vi "Rinocloud_explorer_subVI.vi"() -> ()   [LabVIEW 2013]
uses:
  Rinocloud Library.lvlib
  Rinocloud_global_variable.vi
  Rinocloud API endpoint VIs/API_endpoint_subVIs/State_Control.ctl
panel:
  in  "System state":T1={"Active items"={"Active file ID"="", "Active dir ID"="", "Active object ID"="", "Recent ID"="", "Active item:"="<folder> home (id=)", "Source item"="", "Destination item"="", "Source ID"="", "Destination ID"=""}, "Trees"={"Ancestors"=refnum, "Children"=refnum, "Metadata"=refnum}, "New metadata"={"Name"="", "Tags"="", "Notes"="", "Custom metadata"=[]}, "Communication"={"HTTP headers"="", "HTTP body"="", "Project name"="", "User"="", "HTTP ch body"=""}, "Controls"={"Move refnum"=refnum}, "Status messages"={"error "={"status"=FALSE, "code"=0, "source"=""}, "status"=""}, "Update metadata"={"Name"="", "Tags"="", "Notes"=""}, "Pagination"={"total"=0.0, "limit"=0.0, "offset"=0.0, "count"=0.0, " next page refnum"=refnum, "previous page refnum"=refnum, "page indicator"=""}} {"New metadata"."Custom metadata"."Data type" items=["Numeric", "String", "1D array of strings", "1D array of doubles", "Data JSON string", "<null>"]}
  in  "Rino status control":T2={"Navigation controls"={"full path tree"=refnum, "folder content tree"=refnum, "next page"=refnum, "previous page"=refnum, "refresh file list"=refnum, "delete"=refnum, "page indicator string"=refnum}, "New Folder controls"={"next folder"=refnum, "name"="", "tags"="", "notes"="", "metadata array"=[]}, "Upload File controls"={"upoad file"=refnum, "name"="", "tags"="", "notes"="", "metadata array"=[], "Store data locally"=TRUE, "Store metadata locally"=FALSE, "Path Refnum"=refnum}, "Metadata management controls"={"get metadata"=refnum, "update metadata"=refnum, "name"=refnum, "tags"=refnum, "notes"=refnum, "metadata tree"=refnum}, "Status indicators"={"error"=refnum, "active item"=refnum, "last action"=refnum, "http header"=refnum, "http body"=refnum}, "Move file controls"={"source item"=refnum, "destination item"=refnum, "set source"=refnum, "set destination"=refnum, "move"=refnum}} {"Upload File controls"."metadata array"."Data type" items=["Numeric", "String", "1D array of strings", "1D array of doubles", "Data JSON string", "<null>"]; "New Folder controls"."metadata array"."Data type" items=["Numeric", "String", "1D array of strings", "1D array of doubles", "Data JSON string", "<null>"]}
  in  "page indicator":string
  in  "Next page":bool
  in  "Previous page":bool
  out "Last action:":string
  in  "Active item:":string="<folder> home (id=)"
  in  "delete":bool
  in  "refresh list":bool
  in  "Tab Control":T3(tab)=enum."Inspect"
  in  "Cluster 2":T4={"Attribute"="", "Value"="", "Data type"=5} {"Data type" items=["Numeric", "String", "1D array of strings", "1D array of doubles", "Data JSON string", "<null>"]}
  in  "Cluster 1":T4={"Attribute"="", "Value"="", "Data type"=5} {"Data type" items=["Numeric", "String", "1D array of strings", "1D array of doubles", "Data JSON string", "<null>"]}
  in  "name":string
  in  "tags":string
  in  "notes":string
  in  "new folder":bool
  in  "upload file":bool
  in  "Store data locally":bool=TRUE
  in  "Store metadata locally":bool
  in  "Name:":string
  in  "Tags:":string
  in  "Notes:":string
  in  "get metadata":bool
  in  "metadata tree":string(tree) caption="Metadata"
  in  "update metadata":bool
  in  "Move":bool
  in  "Destination:":string
  in  "Source:":string
  in  "set source":bool
  in  "set destination":bool
  out "body":string
  out "headers":string
  in  "error message":string caption="Error:"
  in  "ancestor tree":string(tree)="home" caption="Active path"
  in  "stop":bool
  in  "active child tree":string(tree) caption="File & folder list of the active folder"
  # "Double-click an item to activate"
  # "Custom metadata:"
  # "(tag1,tag2,tag3,...)"
  # "Click the fields to edit"
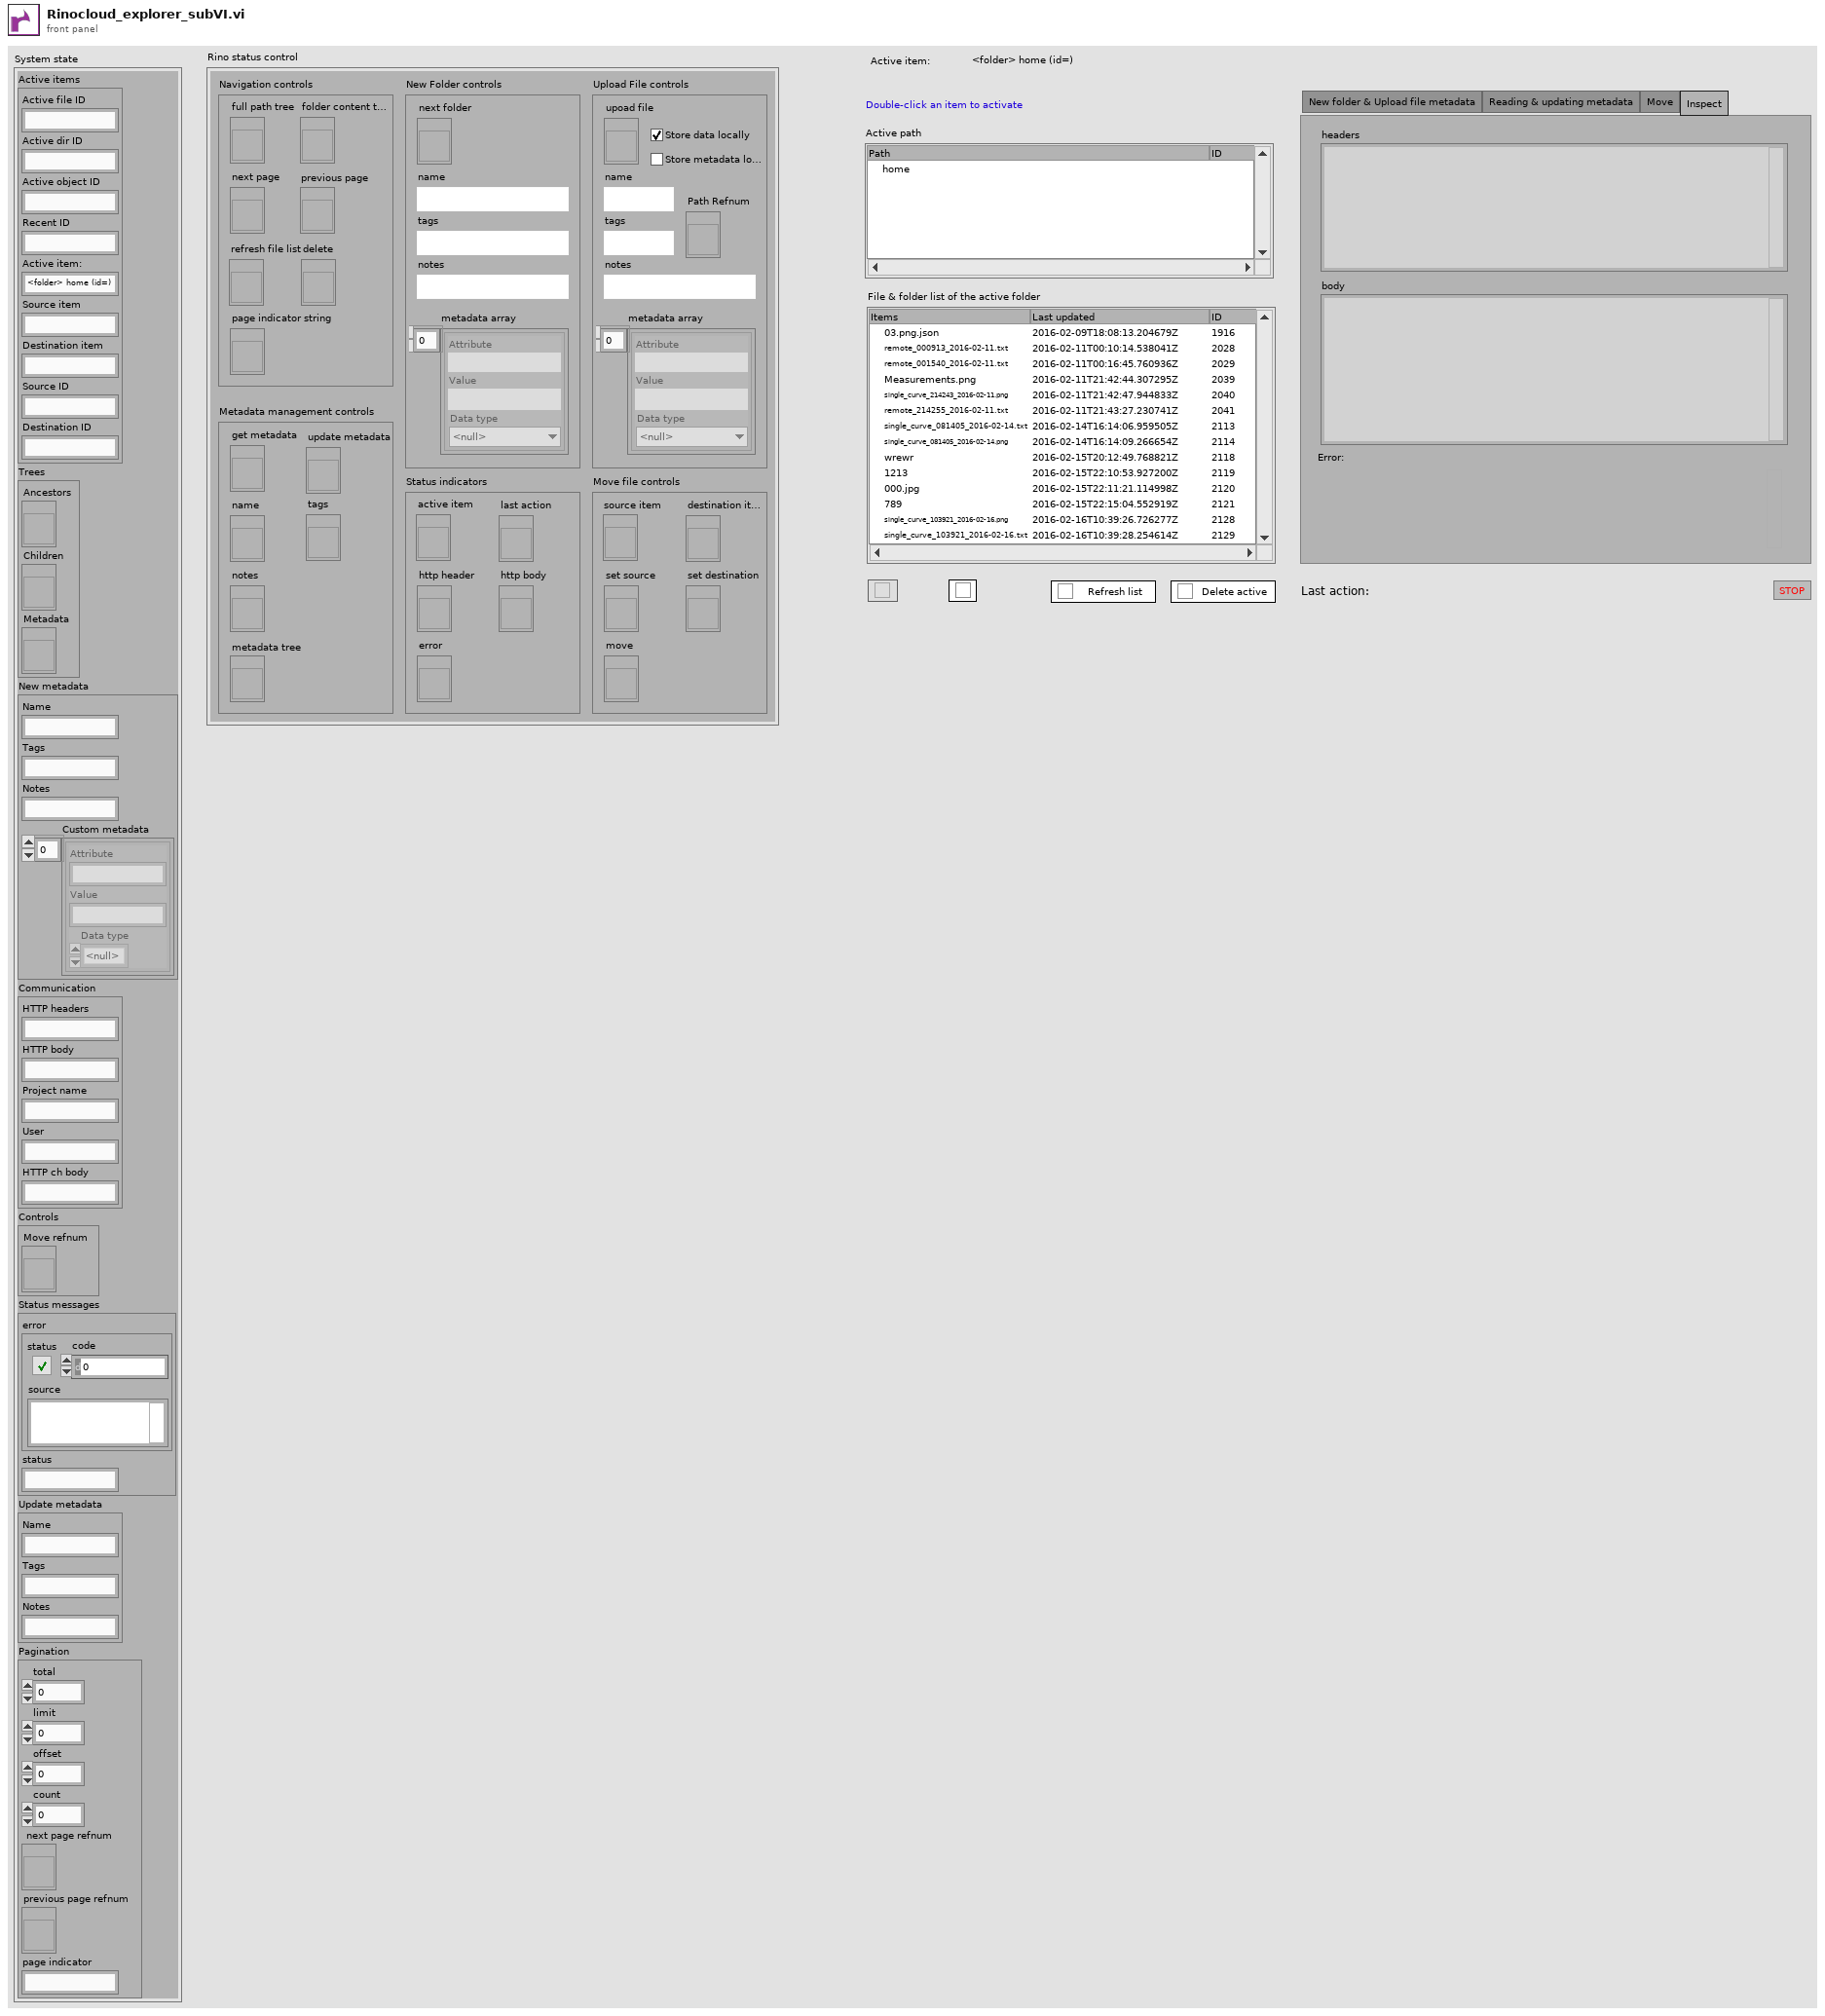
[diagram p1: front panel]
types:
  T1 = cluster{"Active items":cluster{"Active file ID":string, "Active dir ID":string, "Active object ID":string, "Recent ID":string, "Active item:":string, "Source item":string, "Destination item":string, "Source ID":string, "Destination ID":string}, "Trees":cluster{"Ancestors":refnum<vi>, "Children":refnum<vi>, "Metadata":refnum<vi>}, "New metadata":cluster{"Name":string, "Tags":string, "Notes":string, "Custom metadata":cluster{"Attribute":string, "Value":string, "Data type":u16}[]}, "Communication":cluster{"HTTP headers":string, "HTTP body":string, "Project name":string, "User":string, "HTTP ch body":string}, "Controls":cluster{"Move refnum":refnum<vi>}, "Status messages":cluster{"error ":errorcluster, "status":string}, "Update metadata":cluster{"Name":string, "Tags":string, "Notes":string}, "Pagination":cluster{"total":dbl, "limit":dbl, "offset":dbl, "count":dbl, " next page refnum":refnum<vi>, "previous page refnum":refnum<vi>, "page indicator":string}}
  T2 = cluster{"Navigation controls":cluster{"full path tree":refnum<vi>, "folder content tree":refnum<vi>, "next page":refnum<vi>, "previous page":refnum<vi>, "refresh file list":refnum<vi>, "delete":refnum<vi>, "page indicator string":refnum<vi>}, "New Folder controls":cluster{"next folder":refnum<vi>, "name":string, "tags":string, "notes":string, "metadata array":cluster{"Attribute":string, "Value":string, "Data type":u16}[]}, "Upload File controls":cluster{"upoad file":refnum<vi>, "name":string, "tags":string, "notes":string, "metadata array":cluster{"Attribute":string, "Value":string, "Data type":u16}[], "Store data locally":bool, "Store metadata locally":bool, "Path Refnum":refnum<vi>}, "Metadata management controls":cluster{"get metadata":refnum<vi>, "update metadata":refnum<vi>, "name":refnum<vi>, "tags":refnum<vi>, "notes":refnum<vi>, "metadata tree":refnum<vi>}, "Status indicators":cluster{"error":refnum<vi>, "active item":refnum<vi>, "last action":refnum<vi>, "http header":refnum<vi>, "http body":refnum<vi>}, "Move file controls":cluster{"source item":refnum<vi>, "destination item":refnum<vi>, "set source":refnum<vi>, "set destination":refnum<vi>, "move":refnum<vi>}}
  T3 = enum32{"New folder & Upload file metadata", "Reading & updating metadata", "Move", "Inspect"}
  T4 = cluster{"Attribute":string, "Value":string, "Data type":u16}
  T5 = typedef "State_Control.ctl" = enum16{"Boot", "Initialize", "Wait for event", "Refresh", "Pagination", "Metadata to tree", "Stop"}
  T6 = cluster{"HTTP headers":string, "HTTP body":string, "Project name":string, "User":string, "HTTP ch body":string}
  T7 = cluster{"Active file ID":string, "Active dir ID":string, "Active object ID":string, "Recent ID":string, "Active item:":string, "Source item":string, "Destination item":string, "Source ID":string, "Destination ID":string}
  T8 = enum8{"Enabled", "Disabled", "Disabled and Grayed Out"}
  T9 = cluster{"Name":string, "Tags":string, "Notes":string, "Custom metadata":cluster{"Attribute":string, "Value":string, "Data type":u16}[]}
  T10 = enum16{"Boot", "Initialize", "Wait for event", "Refresh", "Pagination", "Metadata to tree", "Stop"}
  T11 = cluster{"Store locally":bool, "ancestor array":cluster{"id":string, "name":string, "created_on":string, "updated_on":string, "tags":string, "notes":string, "record type":string, "metadata (JSON)":string}[], "Store metadata":bool}
  T12 = cluster{"Attribute":string, "Value":string, "Data type":enum16{"Numeric", "String", "1D array of strings", "1D array of doubles", "Data JSON string", "<null>"}}[]
  T13 = cluster{"limit":dbl, "total":dbl, "offset":dbl, "count":dbl}
  T14 = cluster{"headers":string, "body":string, "ID":string, "Saved":bool}
  T15 = cluster{"Attribute":string, "Value":string, "Data type":u16}[]
  T16 = cluster{"id":string, "name":string, "created_on":string, "updated_on":string, "tags":string, "notes":string, "record type":string, "metadata (JSON)":string}[]
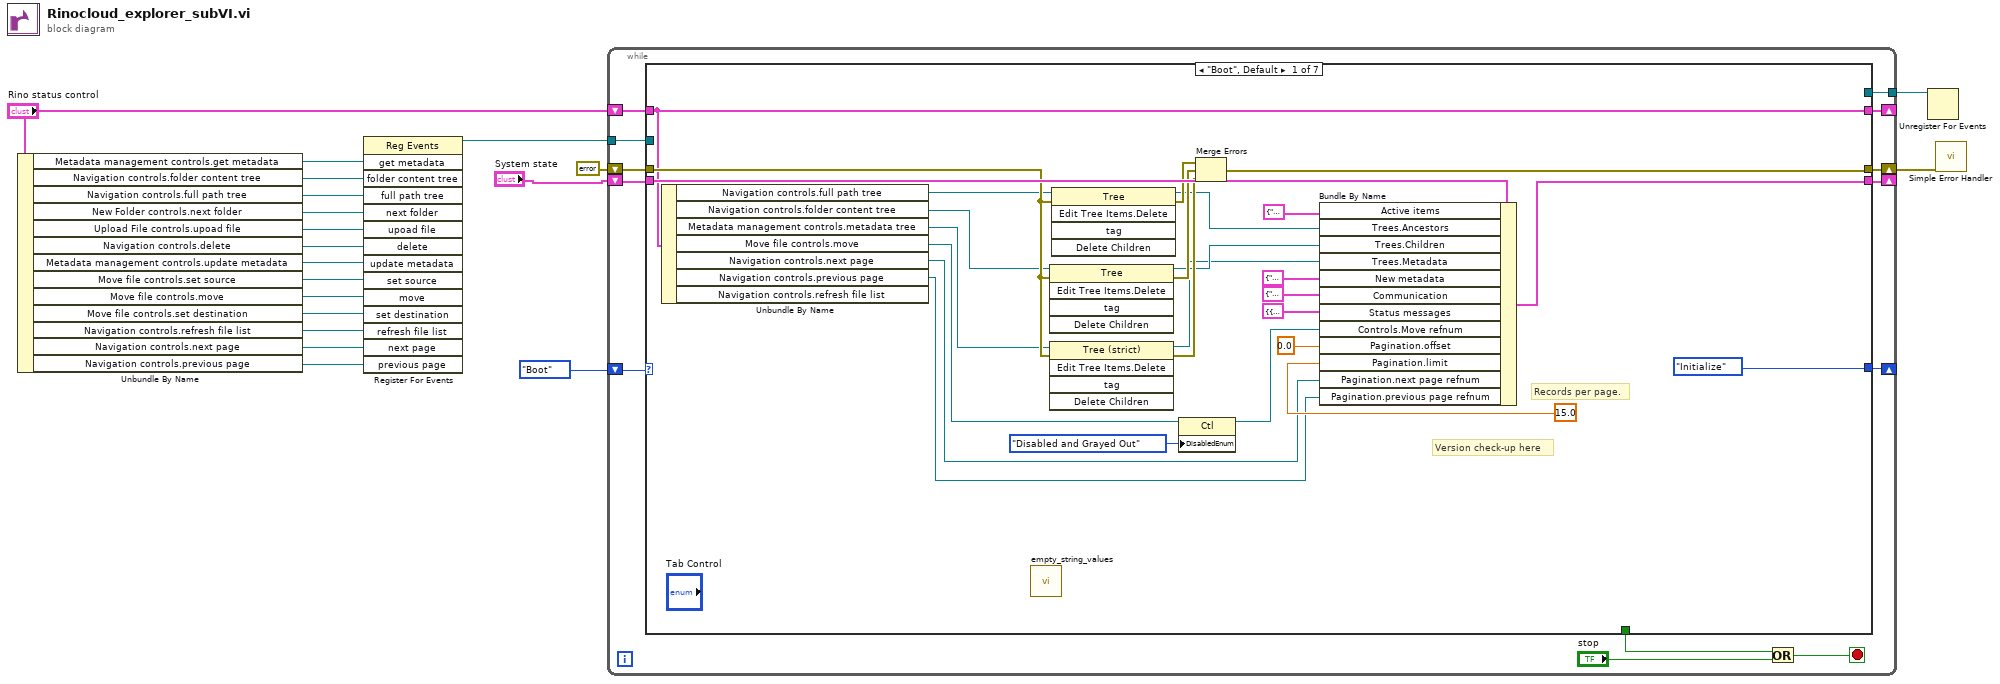
[diagram p0: block diagram]
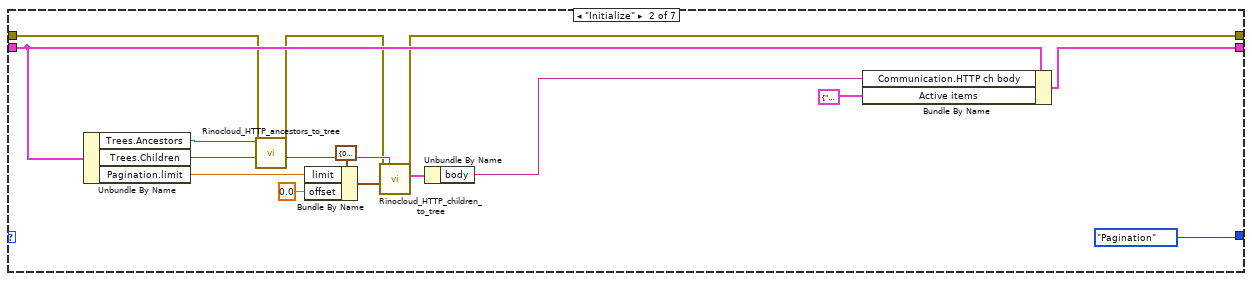
[diagram p2: hidden frame]
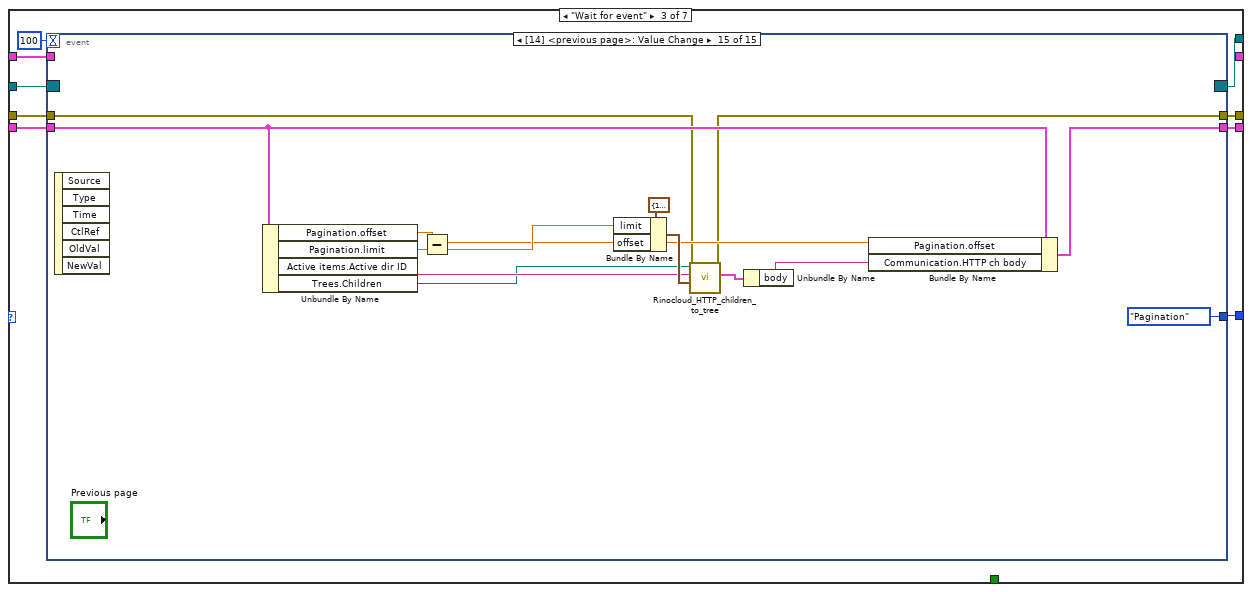
[diagram p3: hidden frame]
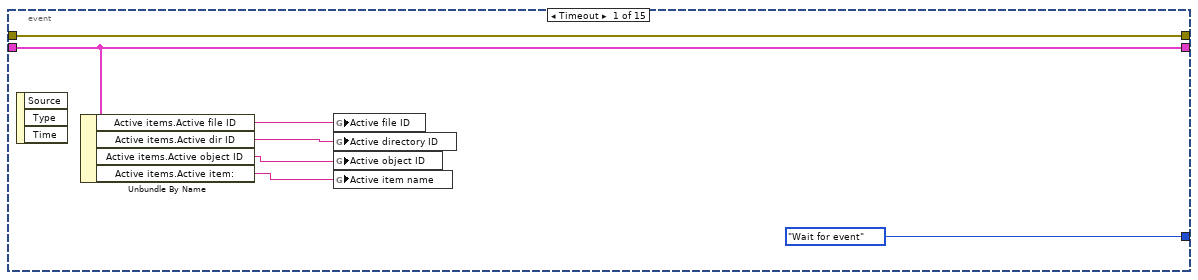
[diagram p4: hidden frame]
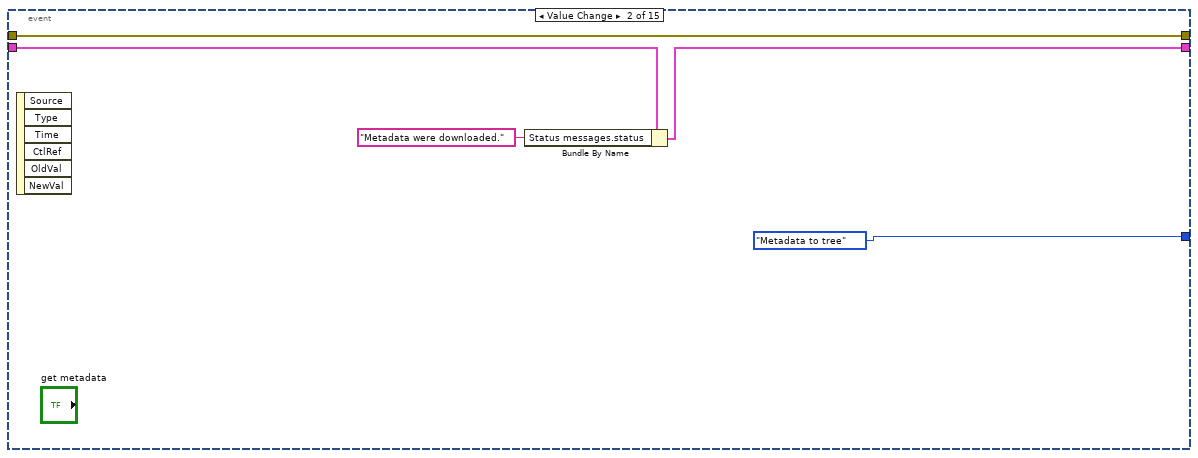
[diagram p5: hidden frame]
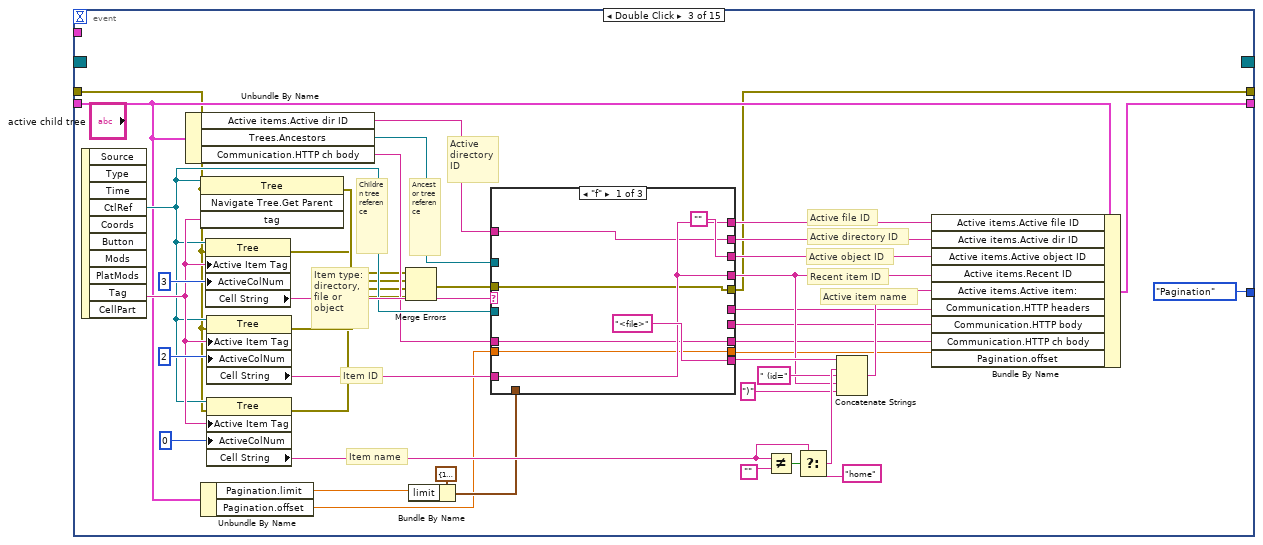
[diagram p6: hidden frame]
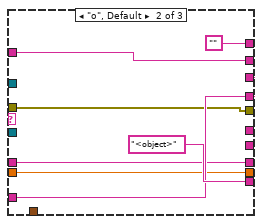
[diagram p7: hidden frame]
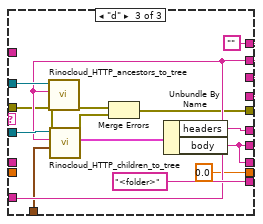
[diagram p8: hidden frame]
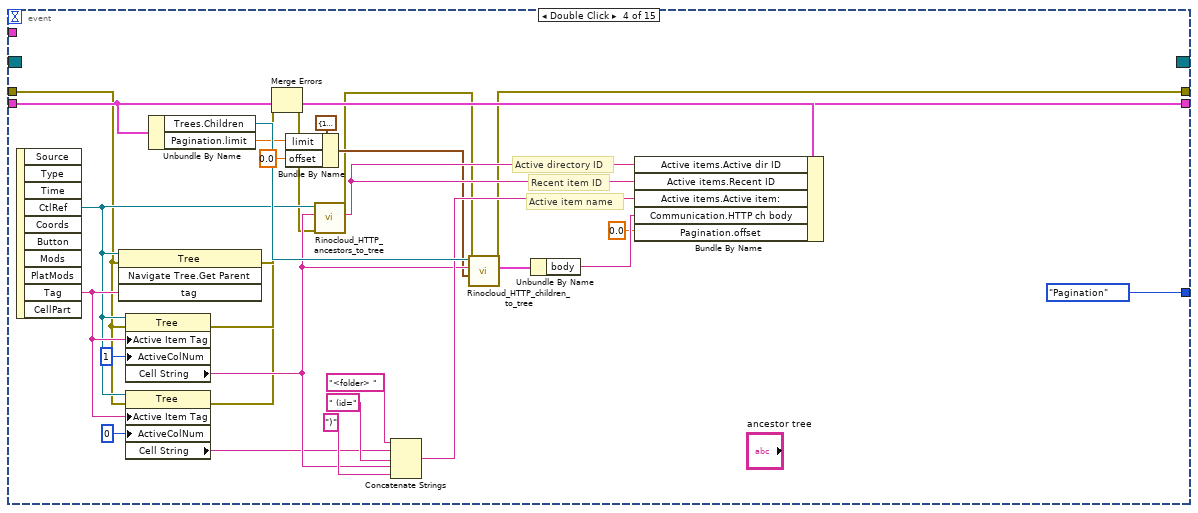
[diagram p9: hidden frame]
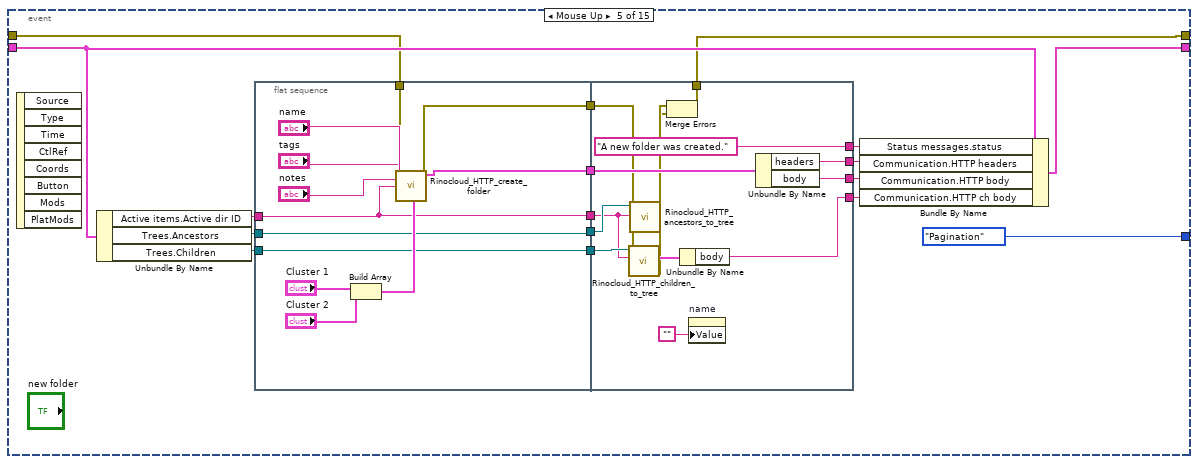
[diagram p10: hidden frame]
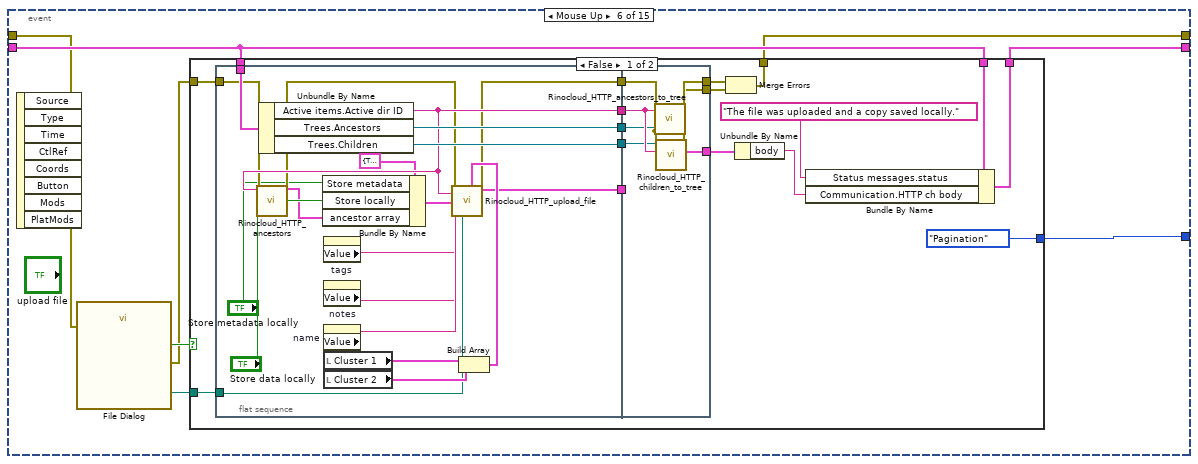
[diagram p11: hidden frame]
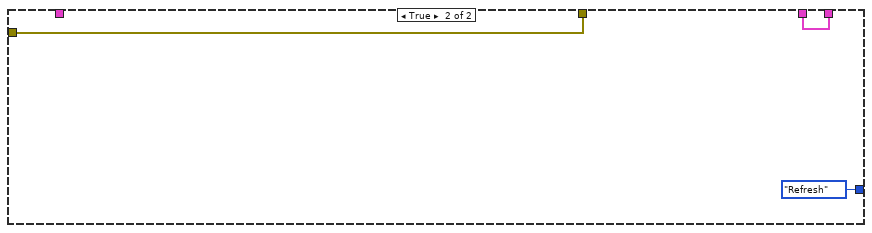
[diagram p12: hidden frame]
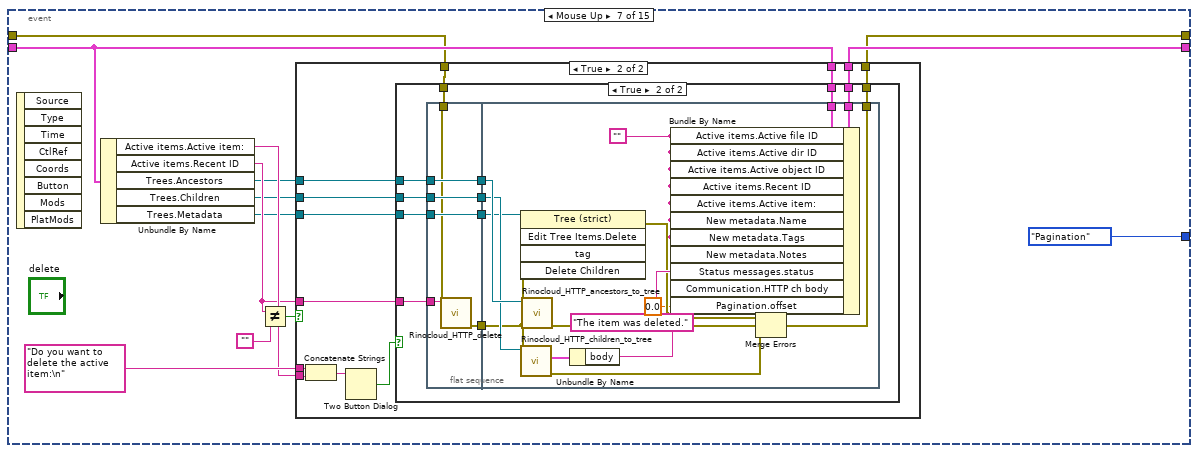
[diagram p13: hidden frame]
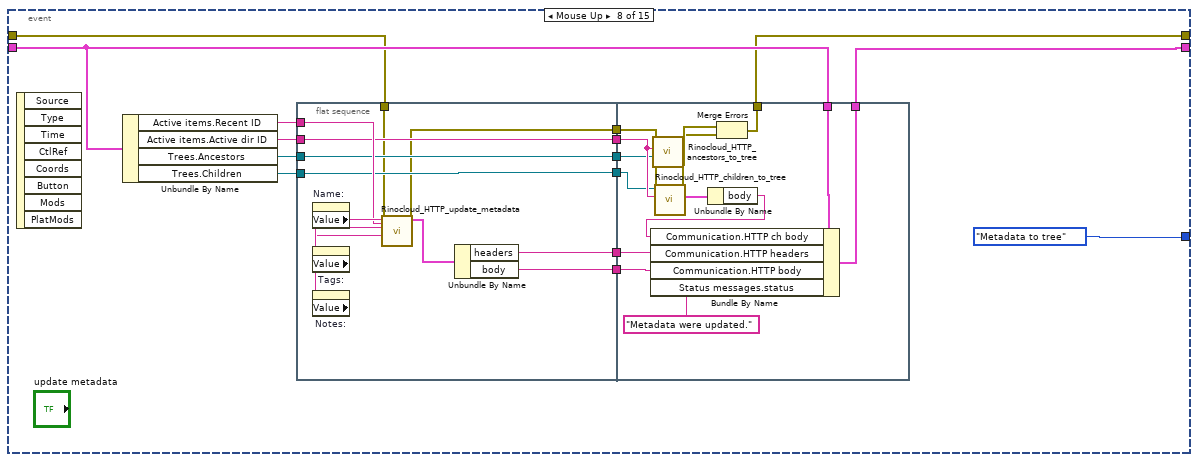
[diagram p16: hidden frame]
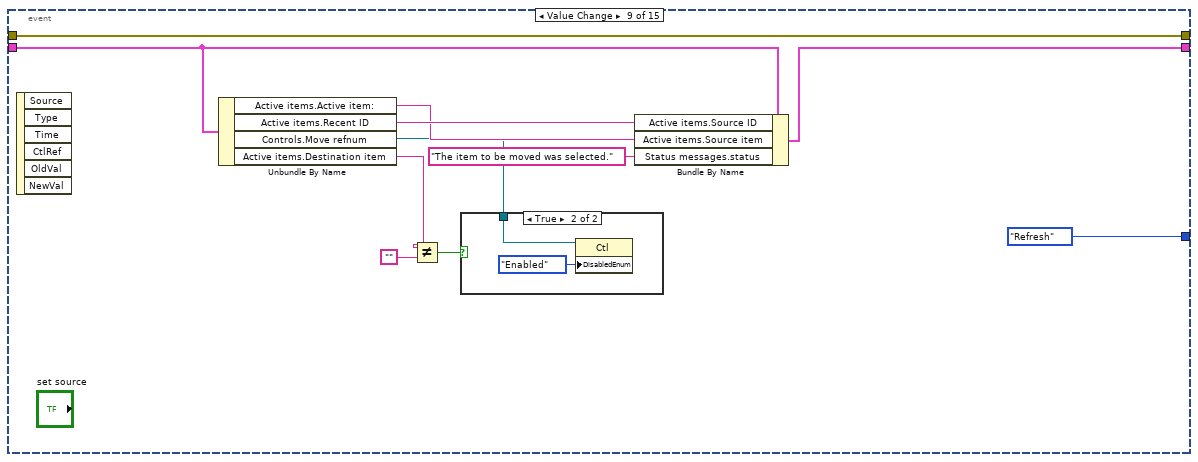
[diagram p17: hidden frame]
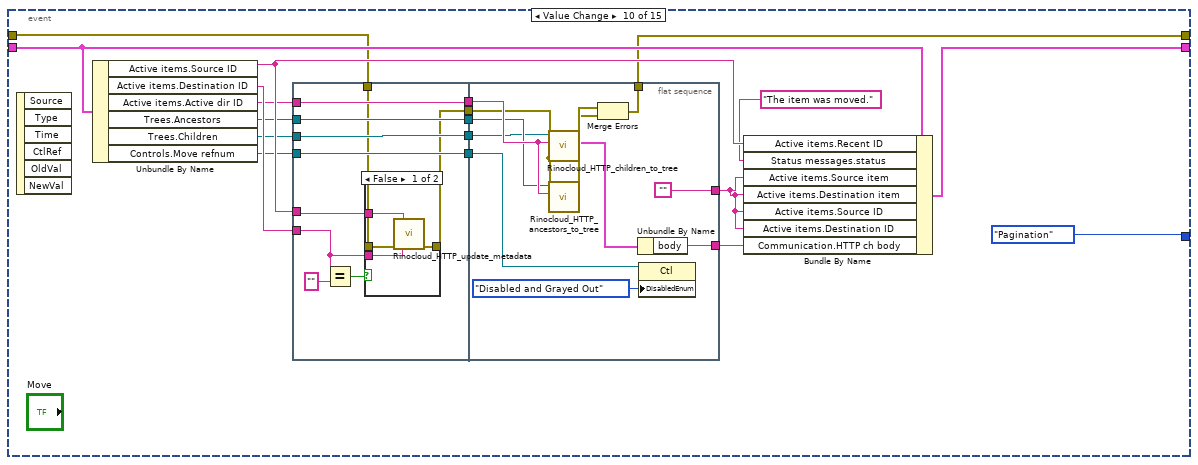
[diagram p19: hidden frame]
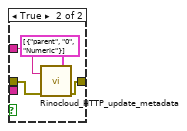
[diagram p20: hidden frame]
diagram:
  n1 = Unbundle By Name("Rino status control") -> ("Metadata management controls.get metadata"=w15:refnum<vi>, "Navigation controls.folder content tree"=w13:refnum<vi>, "Navigation controls.full path tree"=w12:refnum<vi>, "New Folder controls.next folder"=w11:refnum<vi>, "Upload File controls.upoad file"=w10:refnum<vi>, "Navigation controls.delete"=w9:refnum<vi>, "Metadata management controls.update metadata"=w8:refnum<vi>, "Move file controls.set source"=w7:refnum<vi>, "Move file controls.move"=w6:refnum<vi>, "Move file controls.set destination"=w5:refnum<vi>, "Navigation controls.refresh file list"=w4:refnum<vi>, "Navigation controls.next page"=w3:refnum<vi>, "Navigation controls.previous page"=w2:refnum<vi>)
  n2 = register-events(w15, w13, w12, w11, w10, w9, w8, w7, w6, w5, w4, w3, w2) -> (reference out=w17:refnum<event-registration>)  [unwired: 2 in, 1 out]
  n3 = while {
    shift-right: [w27] -> _
    shift-left: State_Control."Boot" -> [w33]
    shift-right: [w28] -> _
    shift-left: "System state" -> [w29]
    shift-right: [w25] -> w18
    shift-left: errorcluster {"status"=FALSE, "code"=0, "source"=""} ("errors") -> [w26]
    tunnel: w17 -> [w24]
    tunnel: [w22] -> w14
    shift-right: [w21] -> _
    shift-left: "Rino status control" -> [w23]
    stop <- w32 stop-if-true
    n4 = case shown="\"Boot\", Default" w33 {
      tunnel: [State_Control."Initialize" T10."Pagination" w82 T10."Wait for event" T10."Metadata to tree" T10."Refresh" T10."Metadata to tree"] -> w27
      tunnel: [_ _ _ _ TRUE _ _] -> w30
      tunnel: w29 -> [w59 w71 w81 w517 w523 w533 w562]
      tunnel: [w56 w70 w80 w517 w523 w532 w561] -> w28
      tunnel: w26 -> [w51 w64 w79 w505 w521 w526 w560]
      tunnel: [w47 w62 w78 _ w521 w525 w559] -> w25
      tunnel: w24 -> [_ _ w77 _ _ _ _]
      tunnel: w23 -> [w37 _ w76 _ _ _ _]
      tunnel: [_ _ w75 _ _ _ _] -> w22
      tunnel: [w37 _ _ _ _ _ _] -> w21
      frame "Boot", Default {
        # "Records per page."
        # "Version check-up here"
        n5 = Unbundle By Name(w37) -> ("Navigation controls.full path tree"=w45:refnum<vi>, "Navigation controls.folder content tree"=w44:refnum<vi>, "Metadata management controls.metadata tree"=w43:refnum<vi>, "Move file controls.move"=w40:refnum<vi>, "Navigation controls.next page"=w39:refnum<vi>, "Navigation controls.previous page"=w38:refnum<vi>)  [unwired: 1 out]
        n6 = call "empty_string_values.vi"() -> ()  [unwired: 12 in]
        n7 = invoke class="Tree" method="Edit Tree Items.Delete"(reference=w44, error in=w51) -> (reference out=w35:refnum<vi>, error out=w49:errorcluster)  [unwired: 3 in, 3 out]
        n8 = invoke class="Tree (strict)" method="Edit Tree Items.Delete"(reference=w43, error in=w51) -> (reference out=w34:refnum<vi>, error out=w48:errorcluster)  [unwired: 3 in, 3 out]
        n9 = invoke class="Tree" method="Edit Tree Items.Delete"(reference=w45, error in=w51) -> (reference out=w36:refnum<vi>, error out=w50:errorcluster)  [unwired: 3 in, 3 out]
        n10 = property class="Ctl"(reference=w40, "DisabledEnum"=T8."Disabled and Grayed Out" ("Disabled")) -> (reference out=w54:refnum<vi>)  [unwired: 1 in, 1 out]
        n11 = Merge Errors(w50, w49, w48) -> (w47:errorcluster)
        n12 = Bundle By Name(cluster=w59, "Active items"=T7 {"Active file ID"="", "Active dir ID"="", "Active object ID"="", "Recent ID"="", "Active item:"="<folder> home (id=)", "Source item"="", "Destination item"="", "Source ID"="", "Destination ID"=""}, "Trees.Ancestors"=w36, "Trees.Children"=w35, "Trees.Metadata"=w34, "New metadata"=T9 {"Name"="", "Tags"="", "Notes"="", "Custom metadata"=[]} ("Metadata"), "Communication"=T6 {"HTTP headers"="", "HTTP body"="", "Project name"="", "User"="", "HTTP ch body"=""}, "Status messages"=cluster{"error ":errorcluster, "status":string} {"error "={"status"=FALSE, "code"=0, "source"=""}, "status"=""}, "Controls.Move refnum"=w54, "Pagination.offset"=0.0, "Pagination.limit"=15.0, "Pagination.next page refnum"=w39, "Pagination.previous page refnum"=w38) -> (w56:T1)
      }
      frame "Initialize" {
        n13 = Unbundle By Name(w71) -> ("Trees.Ancestors"=w72:refnum<vi>, "Trees.Children"=w73:refnum<vi>, "Pagination.limit"=w65:dbl)
        n14 = call "Rinocloud_HTTP_ancestors_to_tree.vi"("error in (no error)"=w64, "Tree Ref in"=w72) -> ("error out"=w63:errorcluster)  [unwired: 2 in, 3 out]
        n15 = Bundle By Name(cluster=cluster{"limit":dbl, "offset":dbl} {"limit"=0.0, "offset"=0.0} ("Pagination variables"), "limit"=w65, "offset"=0.0) -> (w66:cluster{"limit":dbl, "offset":dbl})
        n16 = call "Rinocloud_HTTP_children_to_tree.vi"("error in (no error)"=w63, "Pagination variables"=w66, "Tree Ref in"=w73) -> ("error out"=w62:errorcluster, "Status"=w74:T14)  [unwired: 6 in, 1 out]
        n17 = Unbundle By Name(w74) -> ("body"=w68:string)
        n18 = Bundle By Name(cluster=w71, "Communication.HTTP ch body"=w68, "Active items"=T7 {"Active file ID"="", "Active dir ID"="", "Active object ID"="", "Recent ID"="", "Active item:"="<folder> home (id=)", "Source item"="", "Destination item"="", "Source ID"="", "Destination ID"=""}) -> (w70:T1)
      }
      frame "Wait for event" {
        n19 = event shown="[14] <previous page>: Value Change" {
          selector: w77 -> [_ _ _ _ _ _ _ _ _ _ _ _ _ _ _]
          dyn-events: [_ _ _ _ _ _ _ _ _ _ _ _ _ _ _] -> w75
          timeout: 100 -> [_ _ _ _ _ _ _ _ _ _ _ _ _ _ _]
          tunnel: [T10."Wait for event" T10."Metadata to tree" T10."Pagination" T10."Pagination" T10."Pagination" w237 T10."Pagination" T10."Metadata to tree" T10."Refresh" T10."Pagination" T10."Refresh" T10."Initialize" T10."Stop" T10."Pagination" T10."Pagination"] -> w82
          tunnel: w81 -> [w86 w94 w112 w189 w204 w242 w296 w361 w405 w425 w462 w474 _ w490 w503]
          tunnel: [w86 w93 w123 w187 w203 w241 w295 w358 w398 w416 w459 w473 _ w488 w502] -> w80
          tunnel: w79 -> [w84 w91 w104 w173 w196 w240 w293 w356 w395 w410 w457 w471 _ w478 w492]
          tunnel: [w84 w91 w98 w167 w194 w238 w292 w354 w395 w408 w457 w471 _ w477 w491] -> w78
          tunnel: w76 -> [_ _ _ _ _ _ _ _ _ _ _ _ _ _ _]
          event Timeout {
            n20 = event-data() -> ()  [unwired: 1 in, 3 out]
            n21 = Unbundle By Name(w86) -> ("Active items.Active file ID"=w90:string, "Active items.Active dir ID"=w89:string, "Active items.Active object ID"=w88:string, "Active items.Active item:"=w87:string)
            n22 = global write "Rinocloud_global_variable.vi" "Active file ID"(w90) -> ()
            n23 = global write "Rinocloud_global_variable.vi" "Active directory ID"(w89) -> ()
            n24 = global write "Rinocloud_global_variable.vi" "Active object ID"(w88) -> ()
            n25 = global write "Rinocloud_global_variable.vi" "Active item name"(w87) -> ()
          }
          event Value Change {
            n26 = event-data() -> ()  [unwired: 1 in, 6 out]
            n27 = Bundle By Name(cluster=w94, "Status messages.status"="Metadata were downloaded.") -> (w93:T1)
          }
          event Double Click {
            # "Active \ndirectory\nID"
            # "Ancestor tree \nreference"
            # "Children tree \nreference"
            # "Item name"
            # "Item type:\ndirectory,\nfile or\nobject"
            # "Item ID"
            # "Active item name"
            # "Recent item ID"
            # "Active object ID"
            # "Active directory ID"
            # "Active file ID"
            n28 = event-data() -> ("CtlRef"=w114:refnum<vi>, "Tag"=w119:string)  [unwired: 1 in, 8 out]
            n29 = Unbundle By Name(w112) -> ("Active items.Active dir ID"=w124:string, "Trees.Ancestors"=w125:refnum<vi>, "Communication.HTTP ch body"=w108:string)
            n30 = invoke on="Invoke Node" class="Tree" method="Navigate Tree.Get Parent"(reference=w114, error in=w104, "tag"=w119) -> (error out=w103:errorcluster)  [unwired: 1 in, 3 out]
            n31 = Unbundle By Name(w112) -> ("Pagination.limit"=w110:dbl, "Pagination.offset"=w96:dbl)
            n32 = property on="Property Node" class="Tree"(reference=w114, error in=w104, "Active Item Tag"=w119, "ActiveColNum"=3 ("Active Cell:Active Column Number")) -> (error out=w102:errorcluster, "Cell String"=w118:string)  [unwired: 1 out]
            n33 = property on="Property Node" class="Tree"(reference=w114, error in=w104, "Active Item Tag"=w119, "ActiveColNum"=2 ("Active Cell:Active Column Number")) -> (error out=w101:errorcluster, "Cell String"=w117:string)  [unwired: 1 out]
            n34 = property on="Property Node" class="Tree"(reference=w114, error in=w104, "Active Item Tag"=w119, "ActiveColNum"=0 ("Active Cell:Active Column Number")) -> (error out=w100:errorcluster, "Cell String"=w116:string)  [unwired: 1 out]
            n35 = Merge Errors(w103, w102, w101, w100) -> (w99:errorcluster)
            n36 = Bundle By Name(cluster=cluster{"limit":dbl, "offset":dbl} {"limit"=15.0, "offset"=0.0} ("Pagination variables"), "limit"=w110) -> (w109:cluster{"limit":dbl, "offset":dbl})
            n37 = case shown="\"f\"" w118 {
              tunnel: w117 -> [w141 w149 w160]
              tunnel: ["<file>" ("f") "<object>" ("f") "<folder>" ("f")] -> w133
              tunnel: [w141 w149 w160] -> w127
              tunnel: ["" w149 w163] -> w128
              tunnel: [w141 "" w163] -> w115
              tunnel: [w140 w147 w160] -> w126
              tunnel: w125 -> [_ _ w162]
              tunnel: w114 -> [_ _ w161]
              tunnel: w124 -> [w140 w147 _]
              tunnel: w109 -> [_ _ w159]
              tunnel: w108 -> [w139 w146 _]
              tunnel: [w139 w146 w156] -> w107
              tunnel: [_ _ w156] -> w106
              tunnel: [_ _ w157] -> w105
              tunnel: w99 -> [w138 w145 w155]
              tunnel: [w138 w145 w152] -> w98
              tunnel: [w137 w144 0.0 ("Pagination.offset")] -> w97
              tunnel: w96 -> [w137 w144 _]
              frame "f" {
              }
              frame "o", Default {
              }
              frame "d" {
                w163 = ""
                n38 = call "Rinocloud_HTTP_ancestors_to_tree.vi"("error in (no error)"=w155, "id"=w160, "Tree Ref in"=w162) -> ("error out"=w154:errorcluster)  [unwired: 1 in, 3 out]
                n39 = call "Rinocloud_HTTP_children_to_tree.vi"("error in (no error)"=w155, "Pagination variables"=w159, "id"=w160, "Tree Ref in"=w161) -> ("error out"=w153:errorcluster, "Status"=w158:T14)  [unwired: 5 in, 1 out]
                n40 = Merge Errors(w154, w153) -> (w152:errorcluster)
                n41 = Unbundle By Name(w158) -> ("headers"=w157:string, "body"=w156:string)
              }
            }
            n42 = Not Equal?(x=w116, y="") -> (x != y?=w135:bool)
            n43 = Select(t=w116, s=w135, f="home") -> (s? t:f=w132:string)
            n44 = Concatenate Strings(w133, w132, " (id=" ("string"), w127, ")" ("string")) -> (w129:string)
            n45 = Bundle By Name(cluster=w112, "Active items.Active file ID"=w115, "Active items.Active dir ID"=w126, "Active items.Active object ID"=w128, "Active items.Recent ID"=w127, "Active items.Active item:"=w129, "Communication.HTTP headers"=w105, "Communication.HTTP body"=w106, "Communication.HTTP ch body"=w107, "Pagination.offset"=w97) -> (w123:T1)
          }
          event Double Click {
            # "Active item name"
            # "Recent item ID"
            # "Active directory ID"
            n46 = event-data() -> ("CtlRef"=w180:refnum<vi>, "Tag"=w183:string)  [unwired: 1 in, 8 out]
            n47 = invoke on="Invoke Node" class="Tree" method="Navigate Tree.Get Parent"(reference=w180, error in=w173, "tag"=w183) -> (error out=w172:errorcluster)  [unwired: 1 in, 3 out]
            n48 = property on="Property Node" class="Tree"(reference=w180, error in=w173, "Active Item Tag"=w183, "ActiveColNum"=1 ("Active Cell:Active Column Number")) -> (error out=w171:errorcluster, "Cell String"=w182:string)  [unwired: 1 out]
            n49 = property on="Property Node" class="Tree"(reference=w180, error in=w173, "Active Item Tag"=w183, "ActiveColNum"=0 ("Active Cell:Active Column Number")) -> (error out=w170:errorcluster, "Cell String"=w181:string)  [unwired: 1 out]
            n50 = Unbundle By Name(w189) -> ("Trees.Children"=w190:refnum<vi>, "Pagination.limit"=w176:dbl)
            n51 = Merge Errors(w172, w171, w170) -> (w169:errorcluster)
            n52 = Bundle By Name(cluster=cluster{"limit":dbl, "offset":dbl} {"limit"=15.0, "offset"=0.0} ("Pagination variables"), "limit"=w176, "offset"=0.0) -> (w177:cluster{"limit":dbl, "offset":dbl})
            n53 = call "Rinocloud_HTTP_ancestors_to_tree.vi"("error in (no error)"=w169, "id"=w182, "Tree Ref in"=w180) -> ("error out"=w168:errorcluster, "last ID"=w188:string)  [unwired: 1 in, 2 out]
            n54 = Concatenate Strings("<folder> " ("string"), w181, " (id=" ("string"), w182, ")" ("string")) -> (w186:string)
            n55 = call "Rinocloud_HTTP_children_to_tree.vi"("error in (no error)"=w168, "Pagination variables"=w177, "id"=w182, "Tree Ref in"=w190) -> ("error out"=w167:errorcluster, "Status"=w175:T14)  [unwired: 5 in, 1 out]
            n56 = Unbundle By Name(w175) -> ("body"=w174:string)
            n57 = Bundle By Name(cluster=w189, "Active items.Active dir ID"=w188, "Active items.Recent ID"=w188, "Active items.Active item:"=w186, "Communication.HTTP ch body"=w174, "Pagination.offset"=0.0) -> (w187:T1)
          }
          event Mouse Up {
            n58 = event-data() -> ()  [unwired: 1 in, 8 out]
            n59 = Unbundle By Name(w204) -> ("Active items.Active dir ID"=w210:string, "Trees.Ancestors"=w209:refnum<vi>, "Trees.Children"=w208:refnum<vi>)
            n60 = flat-sequence {
              tunnel: w210 -> [w221]
              tunnel: w209 -> [w220]
              tunnel: w208 -> [w219]
              tunnel: [w221] -> w207
              tunnel: [w220] -> w206
              tunnel: [w219] -> w205
              tunnel: [w218] -> w202
              tunnel: w196 -> [w212]
              tunnel: [w211] -> w195
              tunnel: w207 -> [w233]
              tunnel: w206 -> [w235]
              tunnel: w205 -> [w234]
              tunnel: w202 -> [w232]
              tunnel: [w231] -> w201
              tunnel: [w230] -> w200
              tunnel: ["A new folder was created." ("Status messages.status")] -> w199
              tunnel: [w227] -> w197
              tunnel: w195 -> [w226]
              tunnel: [w223] -> w194
              frame #0 {
                n61 = Build Array("Cluster 1", "Cluster 2") -> (w222:T15)
                n62 = call "Rinocloud_HTTP_create_folder.vi"("Extra metadata array"=w222, "Parent ID"=w221, "error in (no error)"=w212, "Notes"="notes", "Tags"="tags", "Name"="name") -> ("error out"=w211:errorcluster, "Status"=w218:T14)  [unwired: 2 in]
              }
              frame #1 {
                n63 = call "Rinocloud_HTTP_children_to_tree.vi"("error in (no error)"=w226, "id"=w233, "Tree Ref in"=w234) -> ("error out"=w224:errorcluster, "Status"=w228:T14)  [unwired: 6 in, 1 out]
                n64 = call "Rinocloud_HTTP_ancestors_to_tree.vi"("error in (no error)"=w226, "id"=w233, "Tree Ref in"=w235) -> ("error out"=w225:errorcluster)  [unwired: 1 in, 3 out]
                n65 = Merge Errors(w225, w224) -> (w223:errorcluster)
                n66 = Unbundle By Name(w228) -> ("body"=w227:string)
                n67 = property on="name" class="Str"("Value"="") -> ()  [unwired: 2 in, 2 out]
                n68 = Unbundle By Name(w232) -> ("headers"=w231:string, "body"=w230:string)
              }
            }
            n69 = Bundle By Name(cluster=w204, "Status messages.status"=w199, "Communication.HTTP headers"=w201, "Communication.HTTP body"=w200, "Communication.HTTP ch body"=w197) -> (w203:T1)
          }
          event Mouse Up {
            n70 = event-data() -> ()  [unwired: 1 in, 8 out]
            n71 = call "File Dialog"("error in"=w240) -> ("selected path"=w243:path, "cancelled"=w244:bool, "error out"=w239:errorcluster)  [unwired: 11 in, 1 out]
            n72 = case shown="False" w244 {
              tunnel: w243 -> [w261 _]
              tunnel: w242 -> [w260 _]
              tunnel: w242 -> [w255 w291]
              tunnel: [w253 w291] -> w241
              tunnel: w239 -> [w250 w290]
              tunnel: [w246 w290] -> w238
              tunnel: [T10."Pagination" T10."Refresh"] -> w237
              frame False {
                n73 = flat-sequence {
                  tunnel: w261 -> [w279]
                  tunnel: w260 -> [w272]
                  tunnel: [w271] -> w259
                  tunnel: [w270] -> w258
                  tunnel: [w269] -> w257
                  tunnel: [w268] -> w256
                  tunnel: w250 -> [w265]
                  tunnel: [w263] -> w249
                  tunnel: w259 -> [w286]
                  tunnel: w258 -> [w287]
                  tunnel: w257 -> [_]
                  tunnel: w256 -> [w288]
                  tunnel: [w285] -> w252
                  tunnel: w249 -> [w284]
                  tunnel: [w283] -> w248
                  tunnel: [w282] -> w247
                  frame #0 {
                    n74 = Unbundle By Name(w272) -> ("Active items.Active dir ID"=w268:string, "Trees.Ancestors"=w271:refnum<vi>, "Trees.Children"=w270:refnum<vi>)
                    n75 = call "Rinocloud_HTTP_ancestors.vi"("error in (no error)"=w265, "id"=w268) -> ("error out"=w264:errorcluster, "metadata array"=w273:T16)  [unwired: 2 in, 2 out]
                    n76 = Bundle By Name(cluster=T11 {"Store locally"=TRUE, "ancestor array"=[], "Store metadata"=TRUE} ("local storage"), "Store metadata"="Store metadata locally", "Store locally"="Store data locally", "ancestor array"=w273) -> (w266:T11)
                    n77 = property on="tags" class="Str"() -> ("Value"=w277:string)  [unwired: 2 in, 2 out]
                    n78 = property on="notes" class="Str"() -> ("Value"=w276:string)  [unwired: 2 in, 2 out]
                    n79 = property on="name" class="Str"() -> ("Value"=w278:string)  [unwired: 2 in, 2 out]
                    n80 = local read "Cluster 1"() -> (w281:T4)
                    n81 = local read "Cluster 2"() -> (w280:T4)
                    n82 = Build Array(w281, w280) -> (w275:T15)
                    n83 = call "Rinocloud_HTTP_upload_file.vi"("local storage"=w266, "Extra metadata array"=w275, "Path in"=w279, "Parent ID"=w268, "error in (no error)"=w264, "Notes"=w276, "Tags"=w277, "Name"=w278) -> ("error out"=w263:errorcluster, "Status"=w269:T14)  [unwired: 1 in, 1 out]
                  }
                  frame #1 {
                    n84 = call "Rinocloud_HTTP_ancestors_to_tree.vi"("error in (no error)"=w284, "id"=w288, "Tree Ref in"=w286) -> ("error out"=w283:errorcluster)  [unwired: 1 in, 3 out]
                    n85 = call "Rinocloud_HTTP_children_to_tree.vi"("error in (no error)"=w284, "id"=w288, "Tree Ref in"=w287) -> ("error out"=w282:errorcluster, "Status"=w285:T14)  [unwired: 6 in, 1 out]
                  }
                }
                n86 = Merge Errors(w248, w247) -> (w246:errorcluster)
                n87 = Unbundle By Name(w252) -> ("body"=w251:string)
                n88 = Bundle By Name(cluster=w255, "Status messages.status"="The file was uploaded and a copy saved locally.", "Communication.HTTP ch body"=w251) -> (w253:T1)
              }
              frame True {
              }
            }
          }
          event Mouse Up {
            n89 = event-data() -> ()  [unwired: 1 in, 8 out]
            n90 = Unbundle By Name(w296) -> ("Active items.Active item:"=w301:string, "Active items.Recent ID"=w300:string, "Trees.Ancestors"=w299:refnum<vi>, "Trees.Children"=w298:refnum<vi>, "Trees.Metadata"=w297:refnum<vi>)
            n91 = Not Equal?(x=w300, y="") -> (x != y?=w304:bool)
            n92 = case shown="True" w304 {
              tunnel: w300 -> [_ w316]
              tunnel: "Do you want to delete the active item:\n" ("message") -> [_ w315]
              tunnel: w301 -> [_ w314]
              tunnel: w299 -> [_ w313]
              tunnel: w298 -> [_ w312]
              tunnel: w297 -> [_ w311]
              tunnel: w296 -> [w306 w310]
              tunnel: [w306 w309] -> w295
              tunnel: w293 -> [w305 w308]
              tunnel: [w305 w307] -> w292
              frame False {
              }
              frame True {
                n93 = Concatenate Strings(w315, w314) -> (w318:string)
                n94 = Two Button Dialog(message=w318) -> (T button?=w317:bool)  [unwired: 2 in]
                n95 = case shown="True" w317 {
                  tunnel: w316 -> [_ w332]
                  tunnel: w313 -> [_ w330]
                  tunnel: w312 -> [_ w328]
                  tunnel: w311 -> [_ w326]
                  tunnel: w310 -> [w320 w325]
                  tunnel: [w320 w324] -> w309
                  tunnel: w308 -> [w319 w323]
                  tunnel: [w319 w321] -> w307
                  frame False {
                  }
                  frame True {
                    n96 = flat-sequence {
                      tunnel: w332 -> [w338]
                      tunnel: [w337] -> w331
                      tunnel: w330 -> [w337]
                      tunnel: [w336] -> w329
                      tunnel: w328 -> [w336]
                      tunnel: [w335] -> w327
                      tunnel: w326 -> [w335]
                      tunnel: w323 -> [w334]
                      tunnel: [w333] -> w322
                      tunnel: w331 -> [w353]
                      tunnel: w329 -> [w352]
                      tunnel: w327 -> [w351]
                      tunnel: w325 -> [w350]
                      tunnel: [w347] -> w324
                      tunnel: w322 -> [w344]
                      tunnel: [w340] -> w321
                      frame #0 {
                        n97 = call "Rinocloud_HTTP_delete.vi"("error in (no error)"=w334, "ID"=w338) -> ("error out"=w333:errorcluster)  [unwired: 5 in, 1 out]
                      }
                      frame #1 {
                        w349 = ""
                        n98 = invoke class="Tree (strict)" method="Edit Tree Items.Delete"(reference=w351, error in=w344) -> (error out=w343:errorcluster)  [unwired: 3 in, 4 out]
                        n99 = call "Rinocloud_HTTP_children_to_tree.vi"("error in (no error)"=w344, "Tree Ref in"=w352) -> ("error out"=w341:errorcluster, "Status"=w346:T14)  [unwired: 7 in, 1 out]
                        n100 = call "Rinocloud_HTTP_ancestors_to_tree.vi"("error in (no error)"=w344, "Tree Ref in"=w353) -> ("error out"=w342:errorcluster)  [unwired: 2 in, 3 out]
                        n101 = Unbundle By Name(w346) -> ("body"=w345:string)
                        n102 = Bundle By Name(cluster=w350, "Active items.Active file ID"=w349, "Active items.Active dir ID"=w349, "Active items.Active object ID"=w349, "Active items.Recent ID"=w349, "Active items.Active item:"=w349, "New metadata.Name"=w349, "New metadata.Tags"=w349, "New metadata.Notes"=w349, "Status messages.status"="The item was deleted.", "Communication.HTTP ch body"=w345, "Pagination.offset"=0.0) -> (w347:T1)
                        n103 = Merge Errors(w343, w342, w341) -> (w340:errorcluster)
                      }
                    }
                  }
                }
              }
            }
          }
          event Mouse Up {
            n104 = event-data() -> ()  [unwired: 1 in, 8 out]
            n105 = Unbundle By Name(w361) -> ("Active items.Recent ID"=w368:string, "Active items.Active dir ID"=w366:string, "Trees.Ancestors"=w365:refnum<vi>, "Trees.Children"=w362:refnum<vi>)
            n106 = flat-sequence {
              tunnel: w368 -> [w377]
              tunnel: [w376] -> w367
              tunnel: w366 -> [w376]
              tunnel: w365 -> [w375]
              tunnel: [w375] -> w364
              tunnel: [w374] -> w363
              tunnel: w362 -> [w374]
              tunnel: [w372] -> w360
              tunnel: [w371] -> w359
              tunnel: w356 -> [w370]
              tunnel: [w369] -> w355
              tunnel: w367 -> [w394]
              tunnel: w364 -> [w392]
              tunnel: w363 -> [w393]
              tunnel: w361 -> [w391]
              tunnel: w360 -> [w389]
              tunnel: w359 -> [w388]
              tunnel: [w387] -> w358
              tunnel: w355 -> [w384]
              tunnel: [w381] -> w354
              frame #0 {
                n107 = property on="Name:" class="Str"() -> ("Value"=w378:string)  [unwired: 2 in, 2 out]
                n108 = property on="Tags:" class="Str"() -> ("Value"=w380:string)  [unwired: 2 in, 2 out]
                n109 = property on="Notes:" class="Str"() -> ("Value"=w379:string)  [unwired: 2 in, 2 out]
                n110 = call "Rinocloud_HTTP_update_metadata.vi"("self ID"=w377, "error in (no error)"=w370, "Notes"=w379, "Tags"=w380, "Name"=w378) -> ("error out"=w369:errorcluster, "Status"=w373:T14)  [unwired: 5 in]
                n111 = Unbundle By Name(w373) -> ("headers"=w372:string, "body"=w371:string)
              }
              frame #1 {
                n112 = call "Rinocloud_HTTP_ancestors_to_tree.vi"("error in (no error)"=w384, "id"=w394, "Tree Ref in"=w392) -> ("error out"=w383:errorcluster)  [unwired: 1 in, 3 out]
                n113 = call "Rinocloud_HTTP_children_to_tree.vi"("error in (no error)"=w384, "id"=w394, "Tree Ref in"=w393) -> ("error out"=w382:errorcluster, "Status"=w386:T14)  [unwired: 6 in, 1 out]
                n114 = Unbundle By Name(w386) -> ("body"=w385:string)
                n115 = Bundle By Name(cluster=w391, "Communication.HTTP ch body"=w385, "Communication.HTTP headers"=w389, "Communication.HTTP body"=w388, "Status messages.status"="Metadata were updated.") -> (w387:T1)
                n116 = Merge Errors(w383, w382) -> (w381:errorcluster)
              }
            }
          }
          event Value Change {
            n117 = event-data() -> ()  [unwired: 1 in, 6 out]
            n118 = Unbundle By Name(w405) -> ("Active items.Active item:"=w403:string, "Active items.Recent ID"=w404:string, "Controls.Move refnum"=w400:refnum<vi>, "Active items.Destination item"=w401:string)
            n119 = Not Equal?(x=w401, y="") -> (x != y?=w399:bool)
            n120 = case shown="True" w399 {
              tunnel: w400 -> [_ w406]
              frame False {
              }
              frame True {
                n121 = property class="Ctl"(reference=w406, "DisabledEnum"=T8."Enabled" ("Disabled")) -> ()  [unwired: 1 in, 2 out]
              }
            }
            n122 = Bundle By Name(cluster=w405, "Active items.Source ID"=w404, "Active items.Source item"=w403, "Status messages.status"="The item to be moved was selected.") -> (w398:T1)
          }
          event Value Change {
            n123 = event-data() -> ()  [unwired: 1 in, 6 out]
            n124 = Unbundle By Name(w425) -> ("Active items.Source ID"=w424:string, "Active items.Destination ID"=w426:string, "Active items.Active dir ID"=w422:string, "Trees.Ancestors"=w420:refnum<vi>, "Trees.Children"=w418:refnum<vi>, "Controls.Move refnum"=w414:refnum<vi>)
            n125 = flat-sequence {
              tunnel: w424 -> [w434]
              tunnel: w426 -> [w433]
              tunnel: [w432] -> w423
              tunnel: w422 -> [w432]
              tunnel: [w431] -> w421
              tunnel: w420 -> [w431]
              tunnel: [w430] -> w419
              tunnel: w418 -> [w430]
              tunnel: [w429] -> w415
              tunnel: w414 -> [w429]
              tunnel: w410 -> [w428]
              tunnel: [w427] -> w409
              tunnel: w423 -> [w456]
              tunnel: w421 -> [w455]
              tunnel: w419 -> [w454]
              tunnel: w415 -> [w453]
              tunnel: [""] -> w413
              tunnel: [w450] -> w411
              tunnel: w409 -> [w449]
              tunnel: [w446] -> w408
              frame #0 {
                n126 = Equal?(x=w433, y="") -> (x = y?=w435:bool)
                n127 = case shown="False" w435 {
                  tunnel: w434 -> [w440 w444]
                  tunnel: w433 -> [w439 _]
                  tunnel: w428 -> [w438 w442]
                  tunnel: [w437 w441] -> w427
                  frame False {
                    n128 = call "Rinocloud_HTTP_update_metadata.vi"("parent ID"=w439, "self ID"=w440, "error in (no error)"=w438) -> ("error out"=w437:errorcluster)  [unwired: 7 in, 1 out]
                  }
                  frame True {
                    n129 = call "Rinocloud_HTTP_update_metadata.vi"("Extra metadata array"=T12 [{"Attribute"="parent", "Value"="0", "Data type"=enum."Numeric"}], "self ID"=w444, "error in (no error)"=w442) -> ("error out"=w441:errorcluster)  [unwired: 7 in, 1 out]
                  }
                }
              }
              frame #1 {
                n130 = call "Rinocloud_HTTP_children_to_tree.vi"("error in (no error)"=w449, "id"=w456, "Tree Ref in"=w454) -> ("error out"=w448:errorcluster, "Status"=w445:T14)  [unwired: 6 in, 1 out]
                n131 = call "Rinocloud_HTTP_ancestors_to_tree.vi"("error in (no error)"=w449, "id"=w456, "Tree Ref in"=w455) -> ("error out"=w447:errorcluster)  [unwired: 1 in, 3 out]
                n132 = Merge Errors(w448, w447) -> (w446:errorcluster)
                n133 = Unbundle By Name(w445) -> ("body"=w450:string)
                n134 = property class="Ctl"(reference=w453, "DisabledEnum"=T8."Disabled and Grayed Out" ("Disabled")) -> ()  [unwired: 1 in, 2 out]
              }
            }
            n135 = Bundle By Name(cluster=w425, "Active items.Recent ID"=w424, "Status messages.status"="The item was moved.", "Active items.Source item"=w413, "Active items.Destination item"=w413, "Active items.Source ID"=w413, "Active items.Destination ID"=w413, "Communication.HTTP ch body"=w411) -> (w416:T1)
          }
          event Value Change {
            n136 = event-data() -> ()  [unwired: 1 in, 6 out]
            n137 = Unbundle By Name(w462) -> ("Active items.Active item:"=w461:string, "Active items.Active dir ID"=w467:string, "Controls.Move refnum"=w464:refnum<vi>, "Active items.Source item"=w465:string)
            n138 = Not Equal?(x=w465, y="") -> (x != y?=w463:bool)
            n139 = case shown="True" w463 {
              tunnel: w464 -> [_ w468]
              frame False {
              }
              frame True {
                n140 = property class="Ctl"(reference=w468, "DisabledEnum"=T8."Enabled" ("Disabled")) -> ()  [unwired: 1 in, 2 out]
              }
            }
            n141 = Bundle By Name(cluster=w462, "Active items.Destination item"=w461, "Active items.Destination ID"=w467, "Status messages.status"="The destination folder was set.") -> (w459:T1)
          }
          event Mouse Up {
            n142 = event-data() -> ()  [unwired: 1 in, 8 out]
            n143 = Bundle By Name(cluster=w474, "Status messages.status"="The file list view was refreshed.", "Pagination.offset"=0.0) -> (w473:T1)
          }
          event "stop": Value Change {
            n144 = event-data() -> ()  [unwired: 1 in, 6 out]
          }
          event Value Change {
            n145 = event-data() -> ()  [unwired: 1 in, 6 out]
            n146 = Unbundle By Name(w490) -> ("Pagination.limit"=w484:dbl, "Pagination.offset"=w489:dbl, "Active items.Active dir ID"=w486:string, "Trees.Children"=w479:refnum<vi>)
            n147 = Add(x=w484, y=w489) -> (x+y=w483:dbl)
            n148 = Bundle By Name(cluster=cluster{"limit":dbl, "offset":dbl} {"limit"=15.0, "offset"=0.0} ("Pagination variables"), "limit"=w484, "offset"=w483) -> (w482:cluster{"limit":dbl, "offset":dbl})
            n149 = call "Rinocloud_HTTP_children_to_tree.vi"("error in (no error)"=w478, "Pagination variables"=w482, "id"=w486, "Tree Ref in"=w479) -> ("error out"=w477:errorcluster, "Status"=w481:T14)  [unwired: 5 in, 1 out]
            n150 = Unbundle By Name(w481) -> ("body"=w480:string)
            n151 = Bundle By Name(cluster=w490, "Pagination.offset"=w483, "Communication.HTTP ch body"=w480) -> (w488:T1)
          }
          event Value Change {
            n152 = event-data() -> ()  [unwired: 1 in, 6 out]
            n153 = Unbundle By Name(w503) -> ("Pagination.offset"=w504:dbl, "Pagination.limit"=w497:dbl, "Active items.Active dir ID"=w498:string, "Trees.Children"=w493:refnum<vi>)
            n154 = Subtract(x=w504, y=w497) -> (x-y=w496:dbl)
            n155 = Bundle By Name(cluster=cluster{"limit":dbl, "offset":dbl} {"limit"=15.0, "offset"=0.0} ("Pagination variables"), "limit"=w497, "offset"=w496) -> (w499:cluster{"limit":dbl, "offset":dbl})
            n156 = call "Rinocloud_HTTP_children_to_tree.vi"("error in (no error)"=w492, "Pagination variables"=w499, "id"=w498, "Tree Ref in"=w493) -> ("error out"=w491:errorcluster, "Status"=w495:T14)  [unwired: 5 in, 1 out]
            n157 = Unbundle By Name(w495) -> ("body"=w494:string)
            n158 = Bundle By Name(cluster=w503, "Pagination.offset"=w496, "Communication.HTTP ch body"=w494) -> (w502:T1)
          }
        }
      }
      frame "Refresh" {
        n159 = Unbundle By Name(w517) -> ("New metadata.Name"=w511:string, "New metadata.Tags"=w510:string, "New metadata.Notes"=w509:string, "Communication.HTTP headers"=→"headers":string, "Communication.HTTP body"=→"body":string, "Status messages.status"=→"Last action:":string, "Active items.Active item:"=w514:string, "Active items.Source item"=w513:string, "Active items.Destination item"=w512:string, "Pagination.page indicator"=w507:string)
        n160 = Unbundle By Name(w505) -> ("source"=w506:string)
        n161 = local write "error message"(w506) -> ()
        n162 = local write "Name:"(w511) -> ()
        n163 = local write "Tags:"(w510) -> ()
        n164 = local write "Notes:"(w509) -> ()
        n165 = local write "Active item:"(w514) -> ()
        n166 = local write "Source:"(w513) -> ()
        n167 = local write "Destination:"(w512) -> ()
        n168 = local write "page indicator"(w507) -> ()
      }
      frame "Stop" {
        n169 = control-ref of="This VI"() -> (w520:refnum<vi>)
        n170 = invoke class="VI" method="Default Vals.Reinit All"(reference=w520) -> (reference out=w519:refnum<vi>)  [unwired: 2 in, 2 out]
        n171 = Close Reference(reference=w519) -> ()  [unwired: 1 in, 1 out]
      }
      frame "Metadata to tree" {
        n172 = Unbundle By Name(w533) -> ("Active items.Recent ID"=w528:string, "Trees.Metadata"=w541:refnum<vi>)
        n173 = Not Equal?(x=w528, y="") -> (x != y?=w530:bool)
        n174 = Concatenate Strings("Metadata downloaded (id=" ("Communication.Project name"), w528, ")." ("string")) -> (w529:string)
        n175 = case shown="True" w530 {
          tunnel: w541 -> [w545 w555]
          tunnel: [w544 w554] -> w540
          tunnel: [w544 w553] -> w539
          tunnel: [w544 w552] -> w538
          tunnel: [w544 w551] -> w537
          tunnel: [w544 w550] -> w536
          tunnel: [w544 w549] -> _
          tunnel: w529 -> [_ w549]
          tunnel: w528 -> [_ w548]
          tunnel: w526 -> [w543 w547]
          tunnel: [w542 w546] -> w525
          frame False {
            w544 = ""
            n176 = invoke class="Tree (strict)" method="Edit Tree Items.Delete"(reference=w545, error in=w543) -> (error out=w542:errorcluster)  [unwired: 3 in, 4 out]
          }
          frame True {
            n177 = call "Rinocloud_HTTP_metadata_to_tree.vi"("error in (no error)"=w547, "JSON Tree Expanded Reference"=w555, "id"=w548) -> ("error out"=w546:errorcluster, "Notes"=w552:string, "Tags"=w553:string, "Name"=w554:string, "Status"=w556:T14)  [unwired: 3 in, 1 out]
            n178 = Unbundle By Name(w556) -> ("headers"=w551:string, "body"=w550:string)
          }
        }
        n179 = Bundle By Name(cluster=w533, "New metadata.Name"=w540, "New metadata.Tags"=w539, "New metadata.Notes"=w538, "Communication.HTTP headers"=w537, "Communication.HTTP body"=w536) -> (w532:T1)
      }
      frame "Pagination" {
        n180 = Unbundle By Name(w562) -> ("Communication.HTTP ch body"=w570:string, "Pagination.limit"=w564:dbl, "Pagination.offset"=w563:dbl, "Pagination.next page refnum"=w558:refnum<vi>, "Pagination.previous page refnum"=w557:refnum<vi>)
        n181 = call "Rinocloud_pagination.vi"("error in (no error)"=w560, "HTTP body"=w570) -> ("error out"=w559:errorcluster, "pagination parameters"=w567:T13)  [unwired: 2 in]
        n182 = Unbundle By Name(w567) -> ("total"=w566:dbl)
        n183 = Bundle By Name(cluster=T13 {"limit"=15.0, "total"=0.0, "offset"=0.0, "count"=0.0} ("pagination parameters in"), "total"=w566, "limit"=w564, "offset"=w563) -> (w568:T13)
        n184 = call "Rinocloud_pagination_button_state.vi"("previous refnum"=w557, "next refnum"=w558, "pagination parameters in"=w568) -> ("pagination info"=w565:string)  [unwired: 8 in]
        n185 = Bundle By Name(cluster=w562, "Pagination.limit"=w564, "Pagination.offset"=w563, "Pagination.page indicator"=w565) -> (w561:T1)
      }
    }
    n186 = Or(x=w30, y="stop") -> (x .or. y?=w32:bool)
  }
  n187 = Unregister For Events(event registration refnum=w14) -> ()  [unwired: 1 in, 1 out]
  n188 = call <vilib>:"Simple Error Handler.vi"("error in (no error)"=w18) -> ()  [unwired: 4 in, 5 out]
